vi "SAOMM-MicroSlide.vi"() -> ()   [LabVIEW 2011]
uses:
  <vilib>/Instr/_visa.llb/VISA Configure Serial Port (Instr).vi
panel:
  out "read buffer":string
  in  "Ring":u16(ring) items=["Initialisation", "Mise en faisceau", "Mise hors faisceau"]
  in  "Port Number":refnum<visa-resource-name>
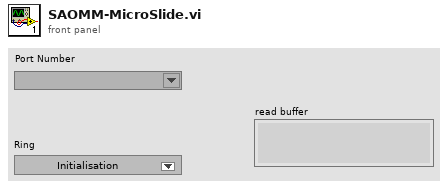
[diagram p1: front panel]
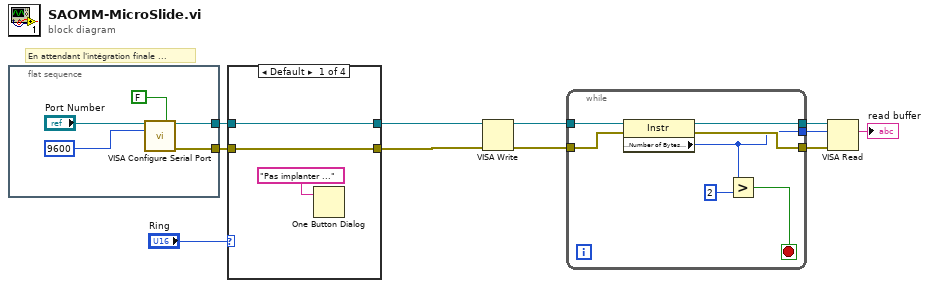
[diagram p0: block diagram]
diagram:
  # "En attendant l'intégration finale ..."
  n1 = flat-sequence {
    tunnel: [w14] -> w10
    tunnel: [w13] -> w9
    frame #0 {
      n2 = call-poly "VISA Configure Serial Port"("VISA resource name"="Port Number", "Enable Termination\nChar (T)"=FALSE ("Enable Termination\nChar (T)"), "baud rate (9600)"=u32 9600) -> ("VISA resource name out"=w14:refnum<visa-resource-name>, "error out"=w13:errorcluster)  [unwired: 11 in]
    }
  }
  n3 = case shown="Default" "Ring" {
    tunnel: w10 -> [w18 w21 _ _]
    tunnel: w9 -> [w17 w20 _ _]
    tunnel: [w18 w21 _ _] -> w4
    tunnel: [w17 w20 _ _] -> w3
    frame Default {
      n4 = One Button Dialog(message="Pas implanter ...") -> ()  [unwired: 1 in, 1 out]
    }
    frame 0 {
    }
    frame 1 {
    }
    frame 2 {
    }
  }
  n5 = VISA Write(VISA resource name=w4, error in (no error)=w3) -> (VISA resource name out=w2:refnum<visa-resource-name>, error out=w1:errorcluster)  [unwired: 1 in, 1 out]
  n6 = while {
    tunnel: w2 -> [w28]
    tunnel: w1 -> [w27]
    tunnel: [w26] -> w5
    tunnel: [w23] -> w6
    tunnel: [w22] -> w7
    stop <- w24 stop-if-true
    n7 = property class="Instr"(reference=w28, error in=w27) -> (reference out=w26:refnum<visa-resource-name>, error out=w23:errorcluster, "Serial Settings:Number of Bytes at Serial Port"=w22:u32)
    n8 = Greater?(x=w22, y=u32 2) -> (0:w24:bool)
  }
  n9 = VISA Read(VISA resource name=w5, byte count=w7, error in (no error)=w6) -> (read buffer=→"read buffer":string)  [unwired: 3 out]
